vi "MS Operation iriss v2.vi"() -> ()   [LabVIEW 2016]
uses:
  <vilib>/Platform/TimedLoop/XDataNode/timing_clust.ctl
  <vilib>/Platform/TimedLoop/XDataNode/nitl_modes.ctl
  <vilib>/Platform/TimedLoop/XDataNode/wakeup.ctl
  Subsystems/Global Variables.vi
  <vilib>/Utility/file.llb/Write Delimited Spreadsheet (DBL).vi
  <vilib>/platform/TimedLoop/XDataNode/XDataNode.xnode
  <vilib>/Platform/TimedLoop/XDataNode/XDNodeRunTimeDep.lvlib
panel:
  in  "file path (dialog if empty)":path=path "D:/Temp Data/delt_rec.csv"
  in  "save data":bool
  out "Free":dbl[](array[numeric])
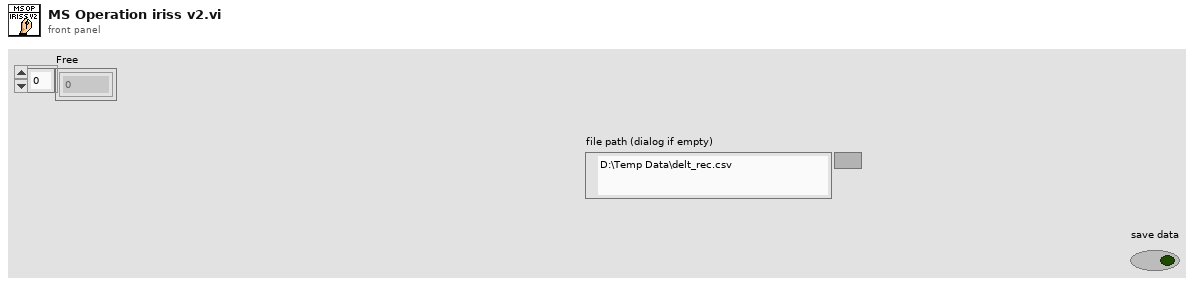
[diagram p1: front panel]
types:
  T1 = typedef "XDNodeRunTimeDep.lvlib/timing_clust.ctl" = cluster{"Expected End [f-1]":u64, "Actual End [f-1]":u64, "Finished Late? [f-1]":bool, "Expected End [i-1]":u64, "Actual End [i-1]":u64, "Finished Late? [i-1]":bool, "Expected Start [i]":u64, "Actual Start [i]":u64, "Expected Start [f]":u64, "Actual Start [f]":u64, "Source Name":string, "Structure Name":string, "Period":i64, "Deadline":i64, "Offset":i64, "Start":i64, "Priority":i32, "Timeout":i32, "Mode":T2, "Wakeup Reason":T3, "Error":errorcluster, "Source Type":string, "Secondary Source Type":string, "Global End Time":u64, "Global Start Time":u64, "Frame Duration":u64, "Iteration Duration":u64, "Assigned CPU":i32, "I/O Scan Engine Mode":u32}
  T2 = typedef "XDNodeRunTimeDep.lvlib/nitl_modes.ctl" = enum32{"No Change", "Process missed periods, maintain original phase", "Discard missed periods, maintain original phase", "Process missed periods, ignore original phase", "Discard missed periods, ignore original phase"}
  T3 = typedef "XDNodeRunTimeDep.lvlib/wakeup.ctl" = enum32{"Normal", "Aborted", "Asynchronous wakeup", "Timing source error", "Timed loop error", "Timeout"}
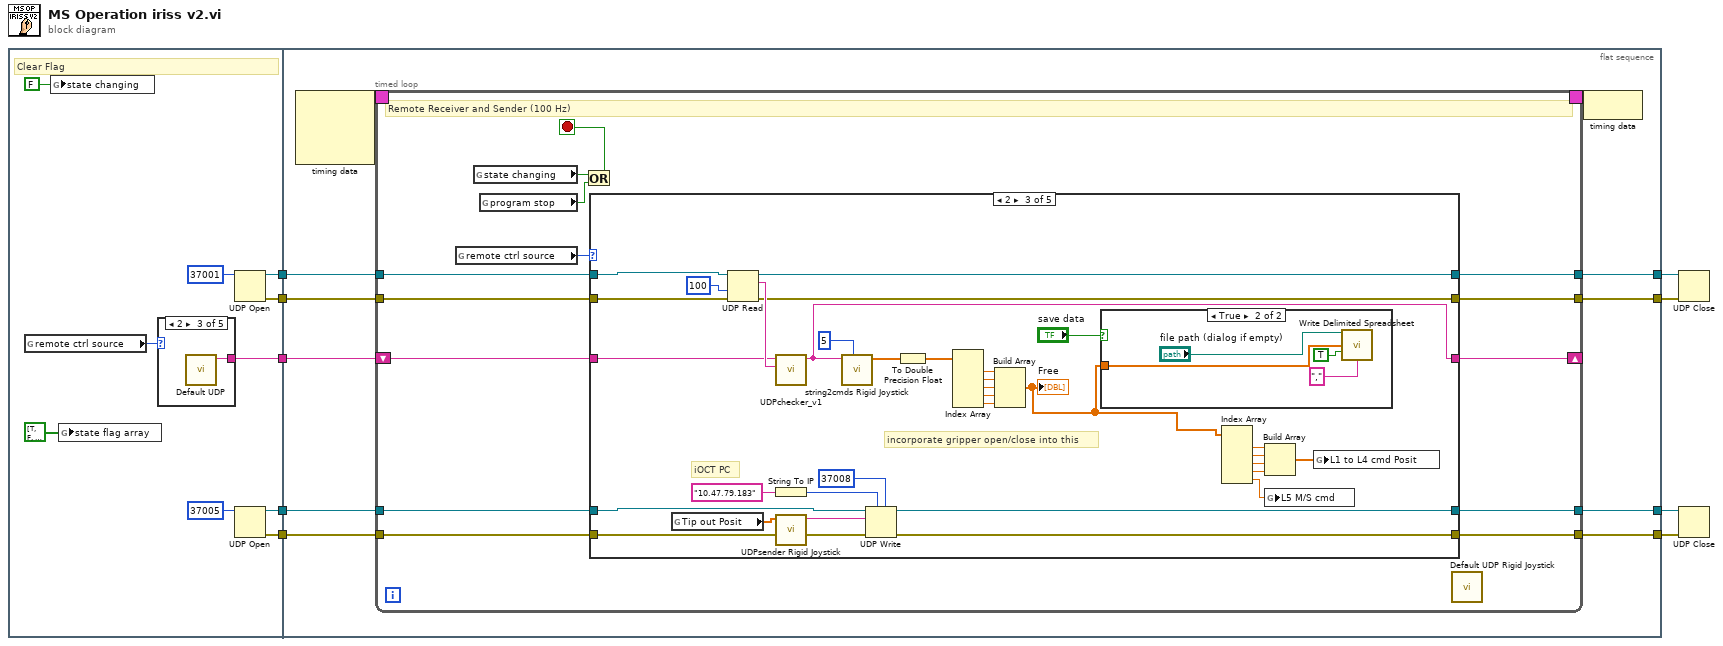
[diagram p0: block diagram]
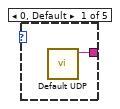
[diagram p2: hidden frame]
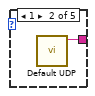
[diagram p3: hidden frame]
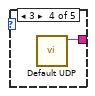
[diagram p4: hidden frame]
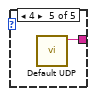
[diagram p5: hidden frame]
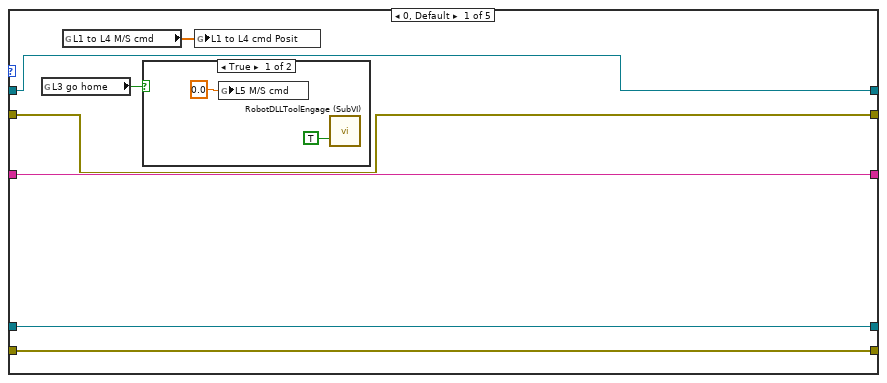
[diagram p6: hidden frame]
diagram:
  n1 = flat-sequence {
    tunnel: [w15] -> w9
    tunnel: [w14] -> w8
    tunnel: [w13] -> w7
    tunnel: [w11] -> w4
    tunnel: [w10] -> w3
    tunnel: w9 -> [w33]
    tunnel: w8 -> [w32]
    tunnel: w7 -> [w31]
    tunnel: [w30] -> w6
    tunnel: [w29] -> w5
    tunnel: w4 -> [w28]
    tunnel: w3 -> [w27]
    tunnel: [w26] -> w2
    tunnel: [w25] -> w1
    frame #0 {
      # "Clear Flag"
      n2 = global read "Global Variables.vi" "remote ctrl source"() -> (w16:u16)
      n3 = global write "Global Variables.vi" "state changing"(FALSE ("state changing")) -> ()
      n4 = global write "Global Variables.vi" "state flag array"(bool[] [TRUE, FALSE, FALSE, FALSE, FALSE, FALSE, FALSE, FALSE, FALSE] ("state flag array")) -> ()
      n5 = case shown="2" w16 {
        tunnel: [w20 w21 w22 w23 w24] -> w14
        frame 0, Default {
          n6 = call "Default UDP.vi"() -> ("String"=w20:string)  [unwired: 11 in]
        }
        frame 1 {
          n7 = call "Default UDP.vi"() -> ("String"=w21:string)  [unwired: 11 in]
        }
        frame 2 {
          n8 = call "Default UDP.vi"() -> ("String"=w22:string)  [unwired: 11 in]
        }
        frame 3 {
          n9 = call "Default UDP.vi"() -> ("String"=w23:string)  [unwired: 11 in]
        }
        frame 4 {
          n10 = call "Default UDP.vi"() -> ("String"=w24:string)  [unwired: 11 in]
        }
      }
      n11 = UDP Open(11:u16 37001 ("port")) -> (port=w13:refnum<k16>, 0:w11:errorcluster)  [unwired: 4 in, 1 out]
      n12 = UDP Open(11:u16 37005 ("port")) -> (port=w15:refnum<k16>, 0:w10:errorcluster)  [unwired: 4 in, 1 out]
    }
    frame #1 {
      n13 = node-c288() -> (w35:T1)  [unwired: 3 in]
      n14 = timed-loop {
        timing: w35 -> [_]
        timing-out: [_] -> w34
        shift-right: [w44] -> _
        shift-left: w32 -> [w45]
        tunnel: w33 -> [w43]
        tunnel: w31 -> [w42]
        tunnel: [w41] -> w30
        tunnel: [w40] -> w29
        tunnel: w28 -> [w39]
        tunnel: w27 -> [w38]
        tunnel: [w37] -> w26
        tunnel: [w36] -> w25
        stop <- w47 stop-if-true
        # "Remote Receiver and Sender (100 Hz)"
        n15 = global read "Global Variables.vi" "remote ctrl source"() -> (w46:u16)
        n16 = global read "Global Variables.vi" "state changing"() -> (w49:bool)
        n17 = global read "Global Variables.vi" "program stop"() -> (w48:bool)
        n18 = Or(x=w49, y=w48) -> (x .or. y?=w47:bool)
        n19 = case shown="2" w46 {
          tunnel: w45 -> [w53 w62 w71 w104 w109]
          tunnel: [w53 w62 w70 w104 w109] -> w44
          tunnel: w43 -> [w54 w63 w75 w105 w110]
          tunnel: w42 -> [w52 w61 w74 w103 w108]
          tunnel: [w54 w63 w73 w105 w110] -> w41
          tunnel: [w52 w61 w72 w103 w108] -> w40
          tunnel: w39 -> [w50 w60 w68 w102 w107]
          tunnel: w38 -> [w51 w59 w67 w101 w106]
          tunnel: [w51 w59 w66 w101 w106] -> w37
          tunnel: [w50 w60 w65 w102 w107] -> w36
          frame 0, Default {
            n20 = global read "Global Variables.vi" "L3 go home"() -> (w56:bool)
            n21 = global read "Global Variables.vi" "L1 to L4 M/S cmd"() -> (w55:dbl[])
            n22 = case shown="True" w56 {
              frame True {
                n23 = global write "Global Variables.vi" "L5 M/S cmd"(0.0 ("L5 M/S cmd")) -> ()
                n24 = call "RobotDLLToolEngage (SubVI).vi"("Tool Fast Retraction"=TRUE ("Tool Withdraw")) -> ()  [unwired: 18 in, 1 out]
              }
              frame False {
              }
            }
            n25 = global write "Global Variables.vi" "L1 to L4 cmd Posit"(w55) -> ()
          }
          frame 1 {
          }
          frame 2 {
            # "incorporate gripper open/close into this"
            # "iOCT PC"
            n26 = global read "Global Variables.vi" "Tip out Posit"() -> (w89:dbl[])
            n27 = UDP Read(connection ID=w74, timeout ms (25000)=100, 8:w68) -> (data out=w95:string, error out=w65:errorcluster, 3:w72:refnum<k16>)  [unwired: 1 in, 2 out]
            n28 = call "UDPchecker_v1.vi"("new string"=w95, "old string"=w71) -> ("output string"=w70:string)  [unwired: 9 in]
            n29 = String To IP(1:"10.47.79.183" ("name")) -> (0:w91:u32)
            n30 = call "UDPsender Rigid Joystick.vi"("nums2send"=w89) -> ("string2send"=w90:string)  [unwired: 10 in]
            n31 = call "string2cmds Rigid Joystick.vi"("numCmds"=5, "input string"=w70) -> ("output cmds"=w94:dbl[])  [unwired: 9 in]
            n32 = UDP Write(address=w91, port or service name=u16 37008, connection ID=w75, data in=w90, 8:w67) -> (error out=w66:errorcluster, 3:w73:refnum<k16>)  [unwired: 1 in]
            n33 = To Double Precision Float(number=w94) -> (double precision float=w87:dbl[])
            n34 = Index Array(array=w87) -> (element #1=w85:dbl, element #2=w86:dbl, element #3=w84:dbl, element #4=w77:dbl, element #5=w76:dbl)  [unwired: 5 in]
            n35 = Build Array(w85, w86, w84, w77, w76) -> (w64:dbl[])
            "Free" <- w64
            n36 = case shown="True" "save data" {
              tunnel: w64 -> [_ w99]
              frame False {
              }
              frame True {
                n37 = call-poly <vilib>:"Write Delimited Spreadsheet.vi"("file path (dialog if empty)"="file path (dialog if empty)", "1D data"=w99, "append to file? (new file:F)"=TRUE, "delimiter (\\t)"="," ("delimiter (\\t)")) -> ()  [unwired: 10 in, 2 out]
              }
            }
            n38 = Index Array(array=w64) -> (element #1=w82:dbl, element #2=w81:dbl, element #3=w80:dbl, element #4=w78:dbl, element #5=w79:dbl)  [unwired: 5 in]
            n39 = Build Array(w82, w81, w80, w78) -> (w83:dbl[])
            n40 = global write "Global Variables.vi" "L5 M/S cmd"(w79) -> ()
            n41 = global write "Global Variables.vi" "L1 to L4 cmd Posit"(w83) -> ()
          }
          frame 3 {
          }
          frame 4 {
          }
        }
        n42 = call "Default UDP Rigid Joystick.vi"() -> ()  [unwired: 11 in, 1 out]
      }
      n43 = node-c288(w34) -> ()
    }
  }
  n44 = UDP Close(connection ID=w5, 8:w1) -> ()  [unwired: 2 out]
  n45 = UDP Close(connection ID=w6, 8:w2) -> ()  [unwired: 2 out]
